vi "mode_resolution.vi"(0 "reference":refnum<class "OSA200.lvclass">, 3 "resolution":u16, 5 "error in (no error)":errorcluster, 7 "ctrl ref":refnum<vi>, 9 "read/write":enum16{"read", "write"}(ring)) -> (14 "duplicate reference":refnum<class "OSA200.lvclass">, 16 "status":string, 17 "resolution out":u16, 19 "error out":errorcluster)   [LabVIEW 2010, in "OSA200.lvclass"]
doc: "Spectral resolution; high resolution mode results in better resolution and lower update rate."
uses:
  OSA200.lvclass
  OSA.lvclass
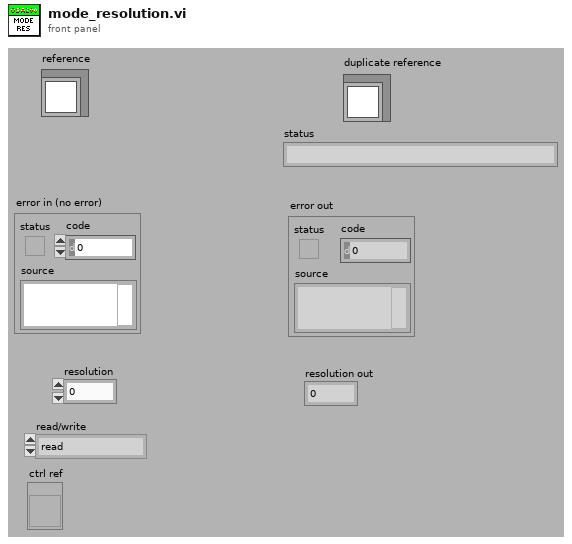
[diagram p1: front panel]
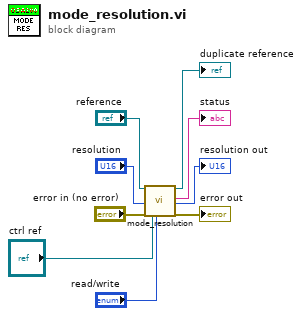
[diagram p0: block diagram]
diagram:
  n1 = call-parent "mode_resolution.vi"("reference"="reference", "resolution"="resolution", "error in (no error)"="error in (no error)", "ctrl ref"="ctrl ref", "read/write"="read/write") -> ("duplicate reference"=→"duplicate reference":refnum<class "OSA200.lvclass">, "status"=→"status":string, "resolution out"=→"resolution out":u16, "error out"=→"error out":errorcluster)  [unwired: 11 in]
